vi "Temperature Reading with add shifter (safe).vi"() -> ()   [LabVIEW 2020]
panel:
  out "Index MIN":dbl
  out "Index MAX":dbl
  out "Temp MIN":dbl
  out "Temp MAX":dbl
  out "WARNING":bool
  in  "stop":bool
  out "Waveform Chart":T1(graph)
  in  "LOW Limit":dbl
  in  "HIGH Limit":dbl
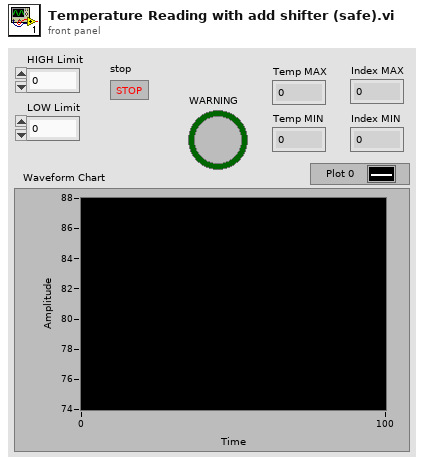
[diagram p1: front panel]
types:
  T1 = cluster{"HIGH Limit":dbl, "Temperature (deg F)":dbl, "LOW Limit":dbl}
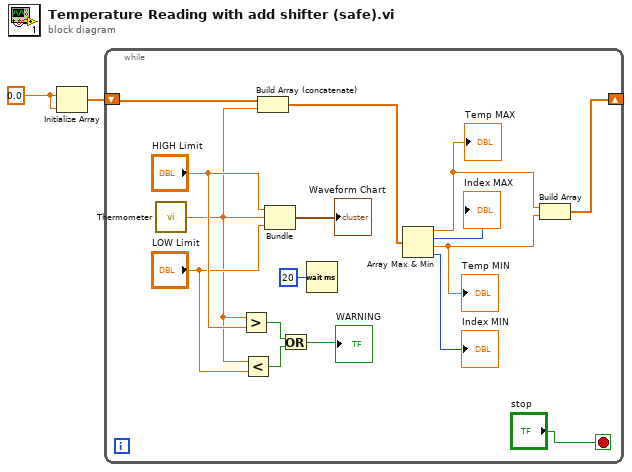
[diagram p0: block diagram]
diagram:
  w2 = 0.0 ("element")
  n1 = Initialize Array "Initialize Array"(w2, w2) -> (w1:dbl[])
  n2 = while {
    shift-right: [w5] -> _
    shift-left: w1 -> [w10]
    stop <- "stop" stop-if-true
    n3 = call "Thermometer.vi"() -> ("Temperature (deg F)"=w9:dbl)  [unwired: 1 in]
    n4 = Greater?(x=w9, y="HIGH Limit") -> (0:w15:bool)
    n5 = Less?(x=w9, y="LOW Limit") -> (x < y?=w14:bool)
    n6 = Build Array (concatenate) "Build Array"(w10, w9) -> (w8:dbl[])
    n7 = Bundle("HIGH Limit"="HIGH Limit", "Temperature (deg F)"=w9, "LOW Limit"="LOW Limit") -> (→"Waveform Chart":T1)  [unwired: 1 in]
    n8 = Or(x=w15, y=w14) -> (x .or. y?=→"WARNING":bool)
    n9 = Wait (ms)(milliseconds to wait=u32 20) -> ()  [unwired: 1 out]
    n10 = Array Max & Min(array=w8) -> (max value=w3:dbl, max index (indices)=→"Index MAX":i32, min value=w4:dbl, min index (indices)=→"Index MIN":i32)
    "Temp MAX" <- w3
    "Temp MIN" <- w4
    n11 = Build Array(w3, w4) -> (w5:dbl[])
  }
